vi "Main.vi"() -> ()   [LabVIEW 2020]
uses:
  WeatherData/WeatherData.lvclass
  CurrentConditionsDisplay/CurrentConditionsDisplay.lvclass
  C:/Projects/Repos/HeadFirstDesignPatterns/HeadFirstDesignPatternsLabVIEWandPython/02 Observer/LabVIEW/DisplayBase/DisplayBase.lvclass
  StatisticsDisplay/StatisticsDisplay.lvclass
  DisplayBase/DisplayBase.lvclass
panel:
  in  "stop":bool
  out "Humidity":dbl(slide) scale=0.0..100.0
  out "Pressure":dbl(slide) scale=0.0..100.0
  out "Temperature":dbl(slide) scale=0.0..100.0
  in  "Generate Data":bool
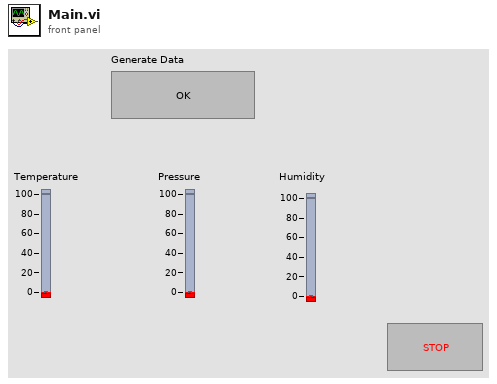
[diagram p1: front panel]
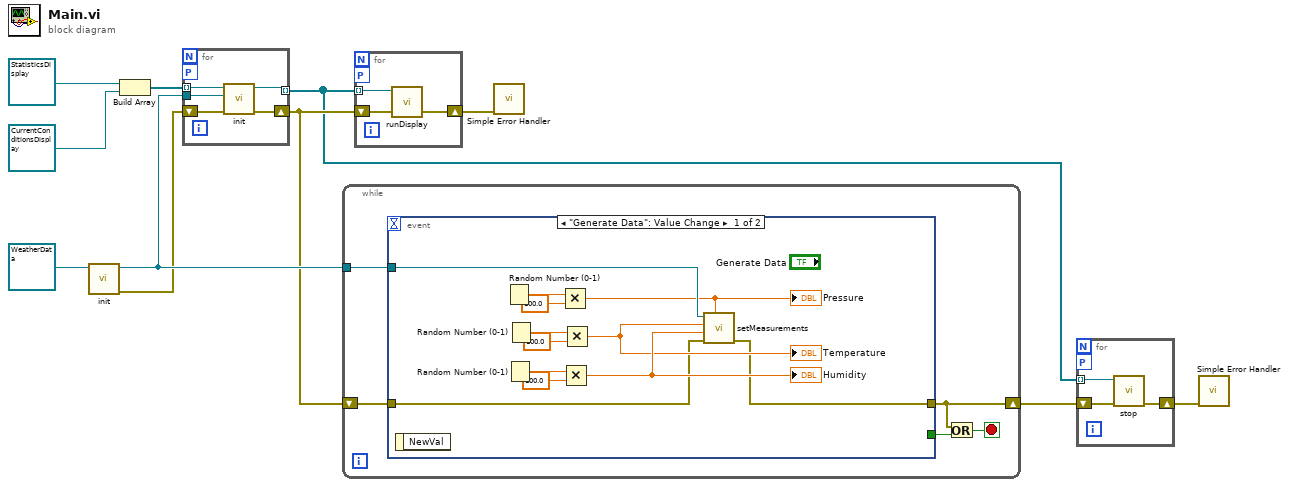
[diagram p0: block diagram]
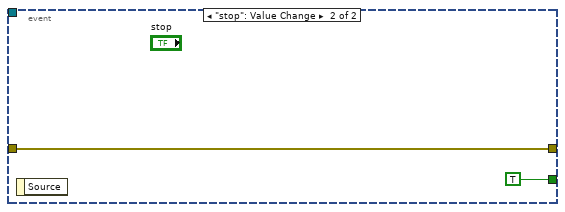
[diagram p2: hidden frame]
diagram:
  n1 = call "init.vi"("WeatherData.lvclass"=refnum<class "WeatherData.lvclass"> refnum) -> ("error out"=w5:errorcluster, "WeatherData.lvclass 2"=w8:refnum<class "WeatherData.lvclass">)  [unwired: 9 in]
  n2 = Build Array(refnum<class "StatisticsDisplay.lvclass"> refnum ("StatisticsDisplay.lvclass"), refnum<class "CurrentConditionsDisplay.lvclass"> refnum ("CurrentConditionsDisplay.lvclass")) -> (w7:refnum<class "DisplayBase.lvclass">[])
  n3 = for {
    tunnel: w7 -> [w16] mode=indexing
    tunnel: [w15] -> w1 mode=indexing
    workers-P: _ -> [_]
    tunnel: w8 -> [w13]
    shift-right: [w14] -> w4
    shift-left: w5 -> [w12]
    n4 = call-dynamic "init.vi"("error in (no error)"=w12, "WeatherData"=w13, "DisplayBase in"=w16) -> ("error out"=w14:errorcluster, "DisplayBase out"=w15:refnum<class "DisplayBase.lvclass">)  [unwired: 7 in]
  }
  n5 = while {
    tunnel: w8 -> [w21]
    shift-right: [w17] -> w3
    shift-left: w4 -> [w19]
    stop <- w18 stop-if-true
    n6 = event shown="[0] \"Generate Data\": Value Change" {
      selector: _ -> [_ _]
      dyn-events: _ -> [_ _]
      timeout: _ -> [_ _]
      tunnel: w21 -> [w27 _]
      tunnel: [_ TRUE ("stop")] -> w20
      tunnel: w19 -> [w23 w34]
      tunnel: [w22 w34] -> w17
      event "Generate Data": Value Change {
        n7 = event-data() -> ()  [unwired: 1 in, 1 out]
        n8 = Random Number (0-1)() -> (number: 0 to 1=w30:dbl)
        n9 = Random Number (0-1)() -> (number: 0 to 1=w28:dbl)
        n10 = Random Number (0-1)() -> (number: 0 to 1=w33:dbl)
        n11 = Multiply(x=w30, y=100.0) -> (x*y=w26:dbl)
        "Pressure" <- w26
        n12 = Multiply(x=w28, y=100.0) -> (x*y=w25:dbl)
        "Humidity" <- w25
        n13 = Multiply(x=w33, y=100.0) -> (x*y=w24:dbl)
        "Temperature" <- w24
        n14 = call "setMeasurements.vi"("Pressure"=w26, "error in (no error)"=w23, "Humidity"=w25, "Temperature"=w24, "WeatherData.lvclass"=w27) -> ("error out"=w22:errorcluster)  [unwired: 5 in, 1 out]
      }
      event "stop": Value Change {
        n15 = event-data() -> ()  [unwired: 1 in, 1 out]
      }
    }
    n16 = Or(x=w17, y=w20) -> (x .or. y?=w18:bool)
  }
  n17 = for {
    tunnel: w1 -> [w38] mode=indexing
    workers-P: _ -> [_]
    shift-right: [w36] -> w6
    shift-left: w4 -> [w37]
    n18 = call-dynamic "runDisplay.vi"("error in (no error)"=w37, "Display"=w38) -> ("error out"=w36:errorcluster)  [unwired: 8 in, 1 out]
  }
  n19 = call <vilib>:"Simple Error Handler.vi"("error in (no error)"=w6) -> ()  [unwired: 4 in, 5 out]
  n20 = for {
    workers-P: _ -> [_]
    shift-right: [w40] -> w2
    shift-left: w3 -> [w41]
    tunnel: w1 -> [w39] mode=indexing
    n21 = call-dynamic "stop.vi"("error in (no error)"=w41, "Display"=w39) -> ("error out"=w40:errorcluster)  [unwired: 8 in, 1 out]
  }
  n22 = call <vilib>:"Simple Error Handler.vi"("error in (no error)"=w2) -> ()  [unwired: 4 in, 5 out]
